vi "Figure.vi"() -> ()   [LabVIEW 2018]
panel:
  in  "Stop (F)":bool
  out "Image Out":T1(plugin-control)
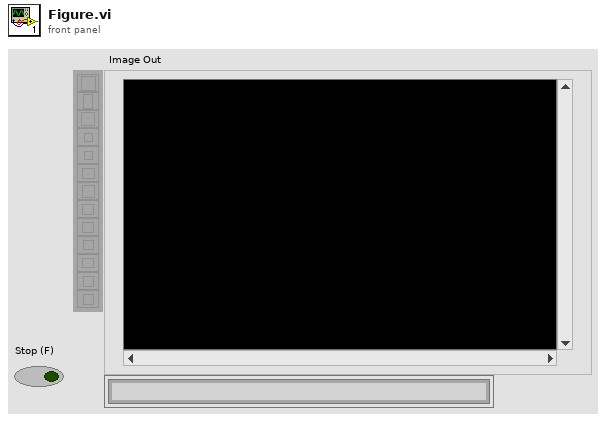
[diagram p1: front panel]
types:
  T1 = typedef "IMAQ Image.ctl" = refnum<image>
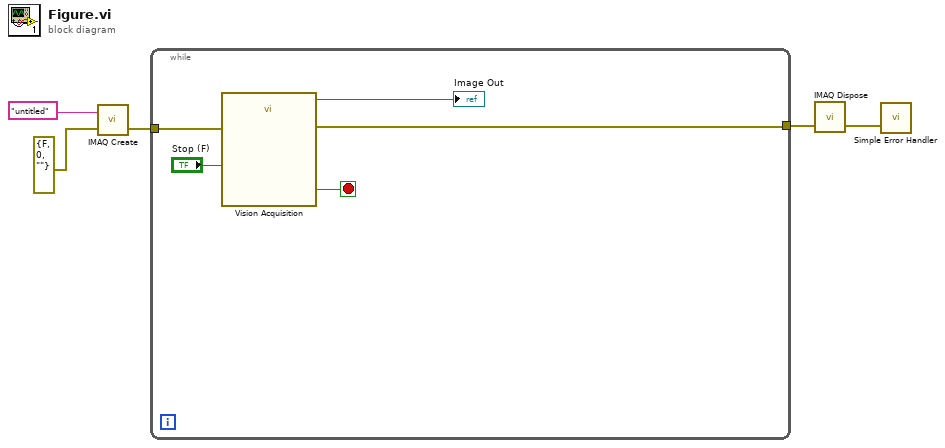
[diagram p0: block diagram]
diagram:
  n1 = call "IMAQ Create"("Image Name"="untitled", "error in (no error)"=errorcluster {"status"=FALSE, "code"=0, "source"=""}) -> ("error out"=w3:errorcluster)  [unwired: 3 in, 1 out]
  n2 = while {
    tunnel: w3 -> [w9]
    tunnel: [w7] -> w2
    stop <- w6 stop-if-true
    n3 = call "Vision Acquisition"("Stop (F)"="Stop (F)", "error in"=w9) -> ("Image Out"=→"Image Out":T1, "Stopped"=w6:bool, "error out"=w7:errorcluster)  [unwired: 23 in]
  }
  n4 = call "IMAQ Dispose"("error in (no error)"=w2) -> ("error out"=w1:errorcluster)  [unwired: 5 in]
  n5 = call <vilib>:"Simple Error Handler.vi"("error in (no error)"=w1) -> ()  [unwired: 4 in, 5 out]
